vi "User32dllAPI.GetWindowText.vi"(8 "error in (no error)":errorcluster, 11 "hWnd":i32) -> (0 "error out":errorcluster, 2 "WindowText":string, 3 "hWnd out":i32)   [LabVIEW 2010]
uses:
  user32.dll
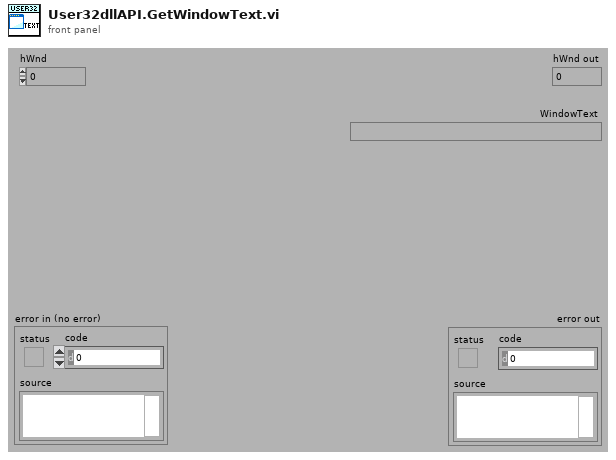
[diagram p1: front panel]
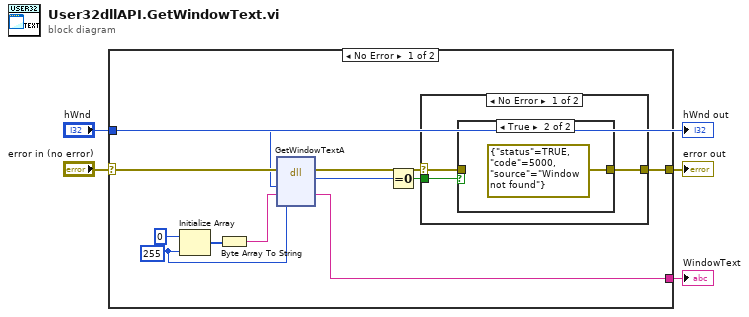
[diagram p0: block diagram]
diagram:
  n1 = case shown="No Error" "error in (no error)" {
    selector: "error in (no error)" -> [w14 w22]
    tunnel: [w12 w22] -> w3
    tunnel: "hWnd" -> [w11 _]
    tunnel: [w6 _] -> w2
    frame No Error {
      w5 = 255 ("length in")
      n2 = Initialize Array(u8 0, w5) -> (w8:u8[])
      n3 = Byte Array To String(unsigned byte array=w8) -> (string=w7:string)
      n4 = dll-call lib="USER32.DLL" fn="GetWindowTextA"(error in=w14, "hwnd"=w11, "lpString"=w7, "nMaxCount"=w5) -> (error out=w13:errorcluster, "result"=w10:i32, "lpString"=w6:string)  [unwired: 4 in, 1 out]
      n5 = Equal To 0?(x=w10) -> (x = 0?=w15:bool)
      n6 = case shown="No Error" w13 {
        selector: w13 -> [w16 w21]
        tunnel: w15 -> [w18 _]
        tunnel: [w17 w21] -> w12
        frame No Error {
          n7 = case shown="True" w18 {
            tunnel: [w19 errorcluster {"status"=TRUE, "code"=5000, "source"="Window not found"} ("error out")] -> w17
            tunnel: w16 -> [w19 _]
            frame False {
            }
            frame True {
            }
          }
        }
        frame Error {
        }
      }
    }
    frame Error {
    }
  }
  "error out" <- w3
  "WindowText" <- w2
  "hWnd out" <- "hWnd"
